vi "Read Time.vi"(8 "error in (no error)":errorcluster, 11 "ControlDragEndedMsg In":refnum<class "ControlDragEndedMsg.lvclass">) -> (0 "error out":errorcluster, 2 "Time":u32, 3 "ControlDragEndedMsg Out":refnum<class "ControlDragEndedMsg.lvclass">)   [LabVIEW 2020, in "MVA Framework.lvlib" / "ActorEvents.lvlib" / "ControlDragEndedMsg.lvclass"]
uses:
  ControlDragEndedMsg.lvclass
  ControlDragEndedMsg.lvclass/ControlDragEndedMsg.ctl
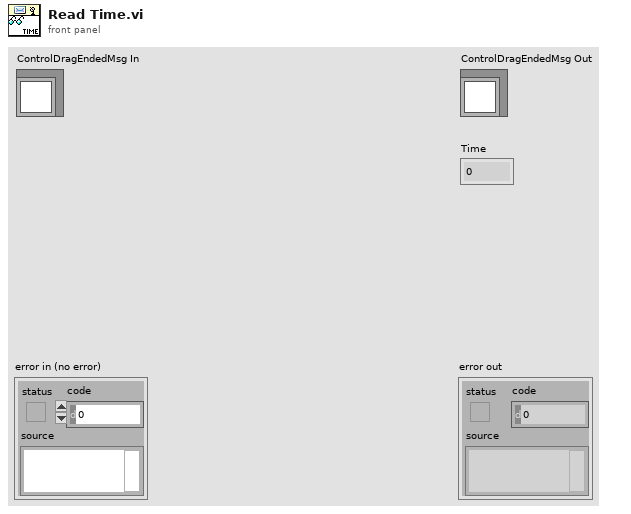
[diagram p1: front panel]
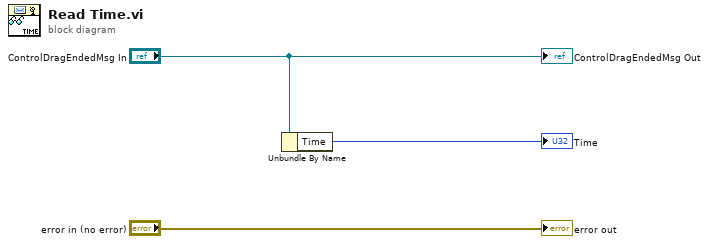
[diagram p0: block diagram]
diagram:
  n1 = Unbundle By Name("ControlDragEndedMsg In") -> ("Time"=→"Time":u32)
  "error out" <- "error in (no error)"
  "ControlDragEndedMsg Out" <- "ControlDragEndedMsg In"
